vi "Global_val_1.vi"() -> ()   [LabVIEW 2022 SP3]
panel:
  out "Ready":bool
  out "Individual processed":bool
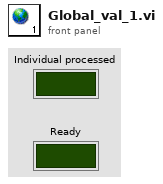
[diagram p1: front panel]
diagram:
